vi "Execute.vi"(8 "error in (no error)":errorcluster, 10 "Abstract Consumer in":refnum<class "Abstract Consumer.lvclass">, 11 "Abstract Request Message in":refnum<class "Abstract Request Message.lvclass">) -> (0 "error out":errorcluster, 1 "Abstract Response out":refnum<class "Abstract Response Message.lvclass">, 2 "Abstract Consumer out":refnum<class "Abstract Consumer.lvclass">, 3 "Abstract Request Message out":refnum<class "Abstract Request Message.lvclass">, 4 "Stop?":bool)   [LabVIEW 2027, in "Messaging.lvlib" / "Abstract Request Message.lvclass"]
uses:
  Abstract Request Message.lvclass
  Consumer/Abstract Consumer/Abstract Consumer.lvclass
  Abstract Response Message/Abstract Response Message.lvclass
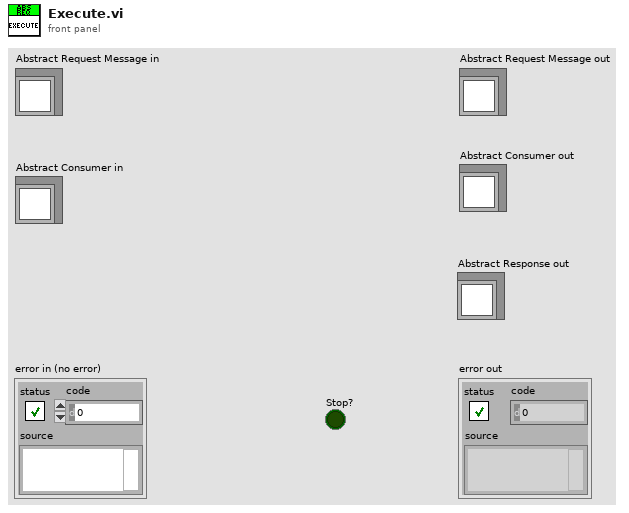
[diagram p1: front panel]
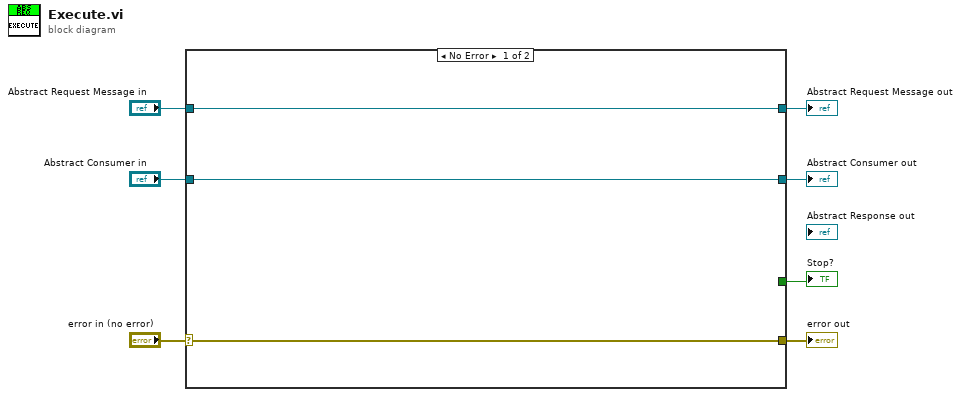
[diagram p0: block diagram]
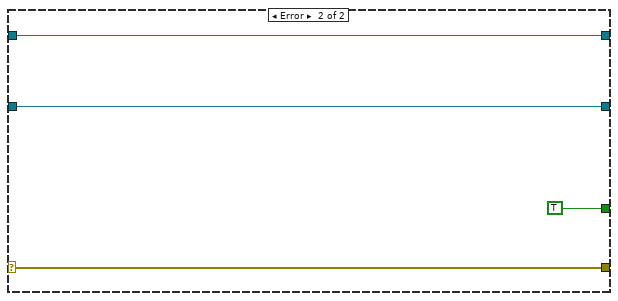
[diagram p2: hidden frame]
diagram:
  n1 = case shown="No Error" "error in (no error)" {
    selector: "error in (no error)" -> [w9 w14]
    tunnel: [w9 w14] -> w6
    tunnel: [w10 w13] -> w4
    tunnel: "Abstract Request Message in" -> [w10 w13]
    tunnel: [w8 w12] -> w3
    tunnel: "Abstract Consumer in" -> [w8 w12]
    tunnel: [_ TRUE ("Stop?")] -> w1
    frame No Error {
    }
    frame Error {
    }
  }
  "error out" <- w6
  "Abstract Request Message out" <- w4
  "Abstract Consumer out" <- w3
  "Stop?" <- w1
